vi "System_Host_2-1-2.vi"() -> ()   [LabVIEW 2017]
uses:
  <vilib>/Analysis/baseanly.llb/Mean (DBL).vi
  <vilib>/Utility/file.llb/Read Delimited Spreadsheet (string).vi
  <vilib>/Utility/file.llb/Write Delimited Spreadsheet (string).vi
  <vilib>/Utility/file.llb/Read Delimited Spreadsheet (DBL).vi
  <vilib>/Utility/file.llb/Write Delimited Spreadsheet (DBL).vi
  <resource>/objmgr/ni.dex.rc
  <vilib>/Analysis/NI_AALBase.lvlib
panel:
  out "System Time [s]":sgl
  out "Power Output":dbl(graph)
  out "Frequency [Hz]":u16(slide) scale=0.0..60.0
  out "Frequency [Hz]":u16(slide) scale=0.0..60.0
  out "Frequency [Hz]":u16(knob) scale=0.0..23.0
  out "Power [W]":dbl(slide) caption="Power Output [W]" scale=0.0..10000.0
  in  "Desired Power [W]":dbl
  out "WT-10":sgl format="%.1g"
  out "BT-11":sgl format="%.1g"
  out "BT-12":sgl format="%.1g"
  out "WT-13":sgl format="%.1g"
  out "CX-10":dbl format="%.1g"
  out "CX-11":dbl format="%.1g"
  out "WT-20":sgl format="%.1f"
  out "BT-21":sgl format="%.1f"
  out "WT-22":sgl format="%.1f"
  out "BT-23":sgl format="%.1f"
  out "WT-24":sgl format="%.1f"
  out "BT-25":sgl format="%.1f"
  out "WT-26":sgl format="%.1f"
  out "BT-27":sgl format="%.1f"
  out "WT-28":sgl format="%.1f"
  out "BT-29":sgl format="%.1f"
  out "BT-30":sgl format="%.1g"
  out "WT-31":sgl format="%.1g"
  out "BT-32":sgl format="%.1g"
  out "WT-33":sgl format="%.1g"
  out "BT-34":sgl format="%.1g"
  out "WT-35":sgl format="%.1g"
  out "WT-40":sgl format="%.1g"
  out "BT-41":sgl format="%.1g"
  out "WT-42":sgl format="%.1g"
  out "BT-43":sgl format="%.1g"
  out "BT-60":sgl format="%.1f"
  out "WT-61":sgl format="%.1f"
  out "WT-62":sgl format="%.1f"
  out "BT-63":sgl format="%.1f"
  out "WT-64":sgl format="%.1f"
  out "BT-65":sgl format="%.1f"
  out "BT-66":sgl format="%.1f"
  out "WT-67":sgl format="%.1f"
  out "ST-10":sgl format="%.1g"
  out "ST-11":sgl format="%.1g"
  out "ST-12":sgl[](array[numeric]) format="%.1g"
  out "ST-13":sgl format="%.1g"
  out "ST-14":sgl[](array[numeric]) format="%.1g"
  out "AT-01":sgl format="%.1g"
  out "AT-02":sgl format="%.1g"
  in  "Power Output On":bool
  in  "Shutdown":bool
  in  "ACTIVATE - CTAH":bool
  in  "CTAH Frequency [Hz]":u16
  in  "ACTIVATE - TCHX":bool
  in  "TCHX Frequency [Hz]":u16
  in  "ACTIVATE - PUMP":bool
  in  "Pump Frequency [Hz]":u16
  out "DHX Primary Flow\n\n\nFM-20 [kg/s]":sgl format="%.3f"
  out "Bypass Flow\n\n\nFM-30 [kg/s]":sgl format="%.3f"
  out "Primary Flow\n\n\nFM-40 [kg/s]":sgl format="%.3f"
  out "DRACS Flow\n\n\nFM-60 [kg/s]":sgl format="%.3f"
  in  "Flow Data?":bool=TRUE
  out "System Safe":bool
  in  "Exit Profile":bool
  in  "Select Operation Mode":T1(ring) caption="Select Operation Mode2"
  out "System Loop Time (ms)":u32
  in  "Load Power Profile":bool
  in  "Dyn. Power Profile File":path
  out "CTAH Temperatures":cluster{"CTAH Outlet":dbl, "CTAH Inlet":dbl}(graph)
  out "CTAH Outlet":dbl format="%0.2f"
  out "CTAH Inlet":dbl format="%0.2f"
  out "Core Temperatures":cluster{"Heater Inlet":dbl, "Heater Outlet":dbl}(graph)
  out "Heater Outlet":dbl format="%0.2f"
  out "Heater Inlet":dbl format="%0.2f"
  out "Profile Step":i32
  out "Power Input Signal [W]":dbl
  out "Output Current 2 [A]":dbl
  out "Output Voltage 2 [V]":dbl
  out "Output Current 1 [A]":dbl
  out "Output Voltage 1 [V]":dbl
  out "Loop Period [ms]":i64
  in  "Pump Operation Mode":i32(listbox)
  in  "TCHX Operation Mode":i32(listbox)
  in  "VFD Stop":bool
  in  "CTAH Operation Mode":i32(listbox)
  in  "Error In":errorcluster
  out "Number of Disconnections":u32
  out "Available Elements for Reading":i32
  out "DAQ?":bool
  in  "Stop DAQ":bool
  out "Error Out":errorcluster
  # "DRACS"
  # "PRIMARY"
  # "HOT DRACS"
  # "HOT LEG"
  # "DHX TOP"
  # "COLD DRACS"
  # "DHX"
  # "BYPASS"
  # "DHX BOTTOM"
  # "COLD LEG"
  # "PUMP"
  # "TCHX"
  # "CTAH"
  # "HEATER"
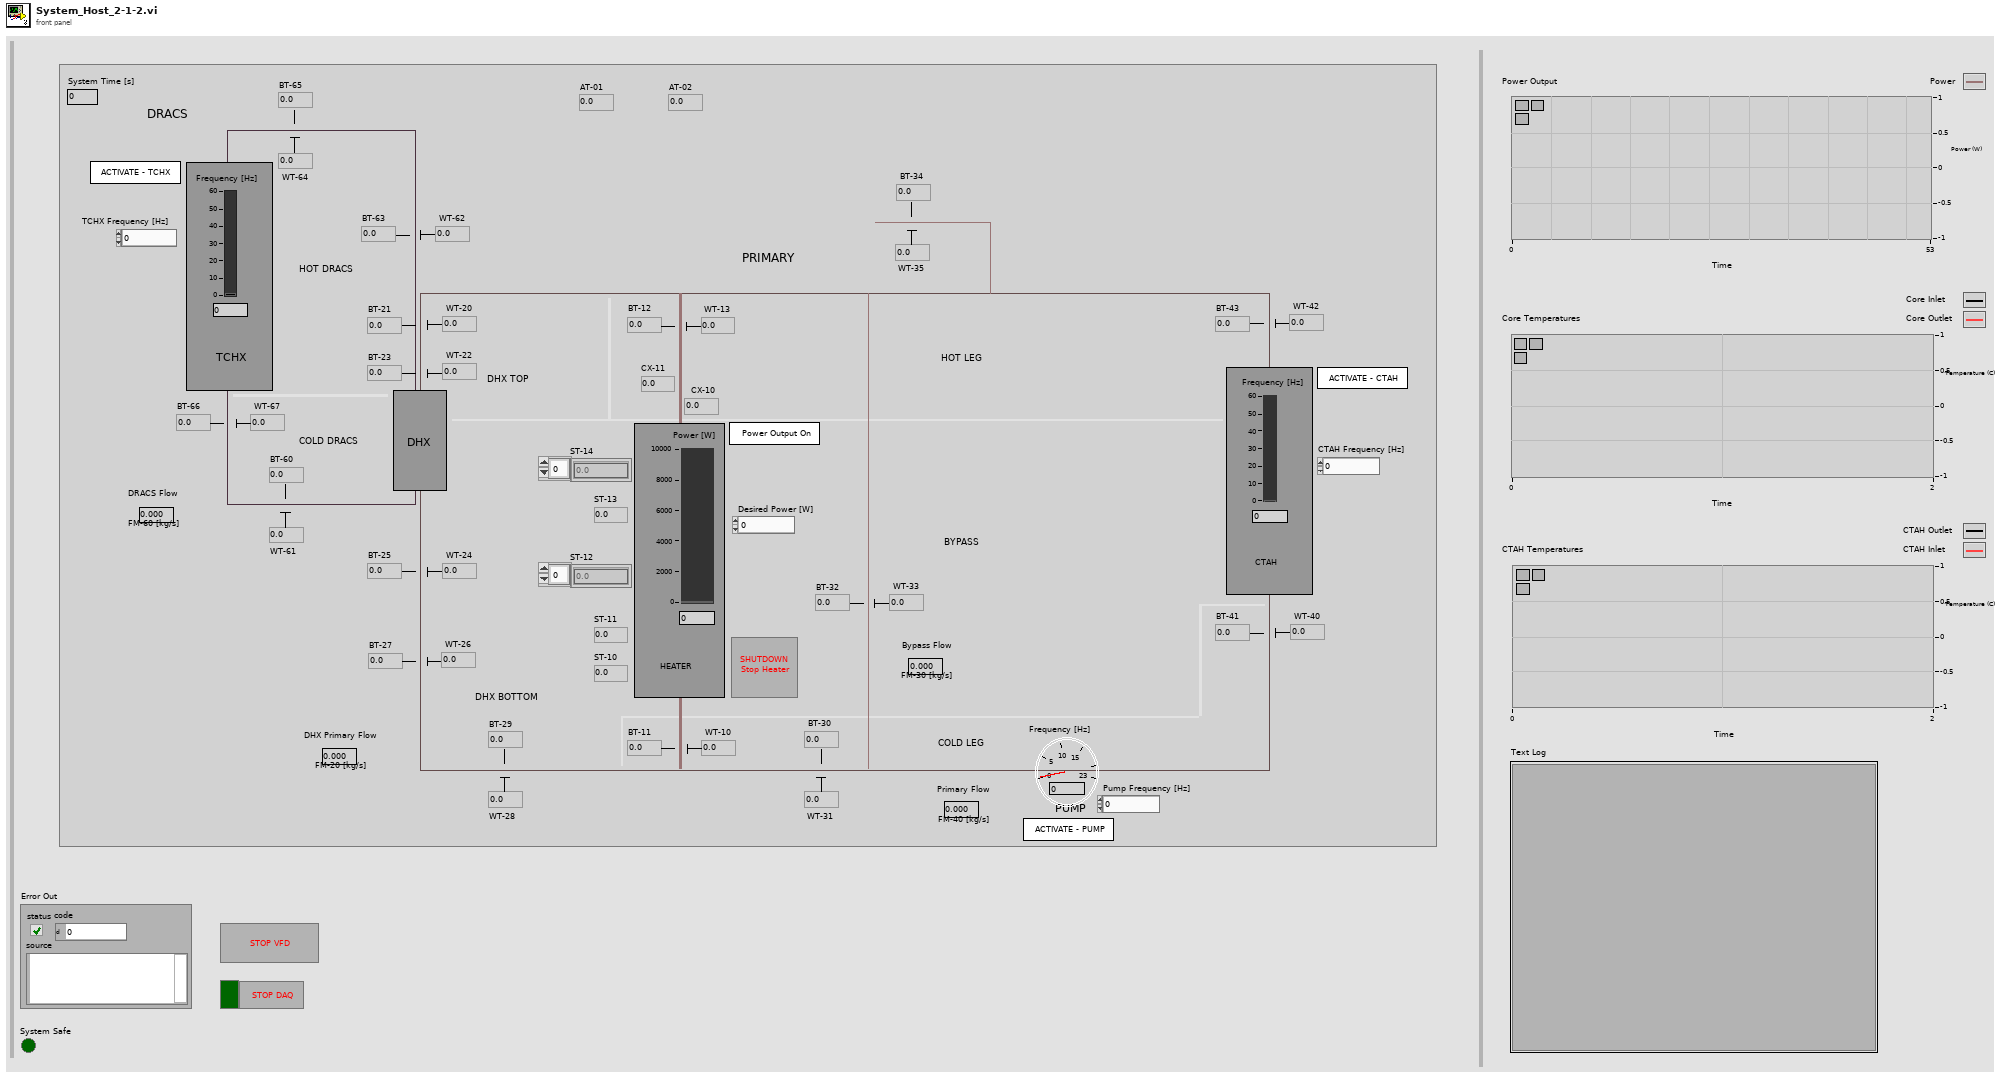
[diagram p1: front panel]
types:
  T1 = enum16{"Resistance Feedback", "Power Profile Input", "Resistance Feedback_Analog", "Power Profile Input_Analog", "Shutdown"}
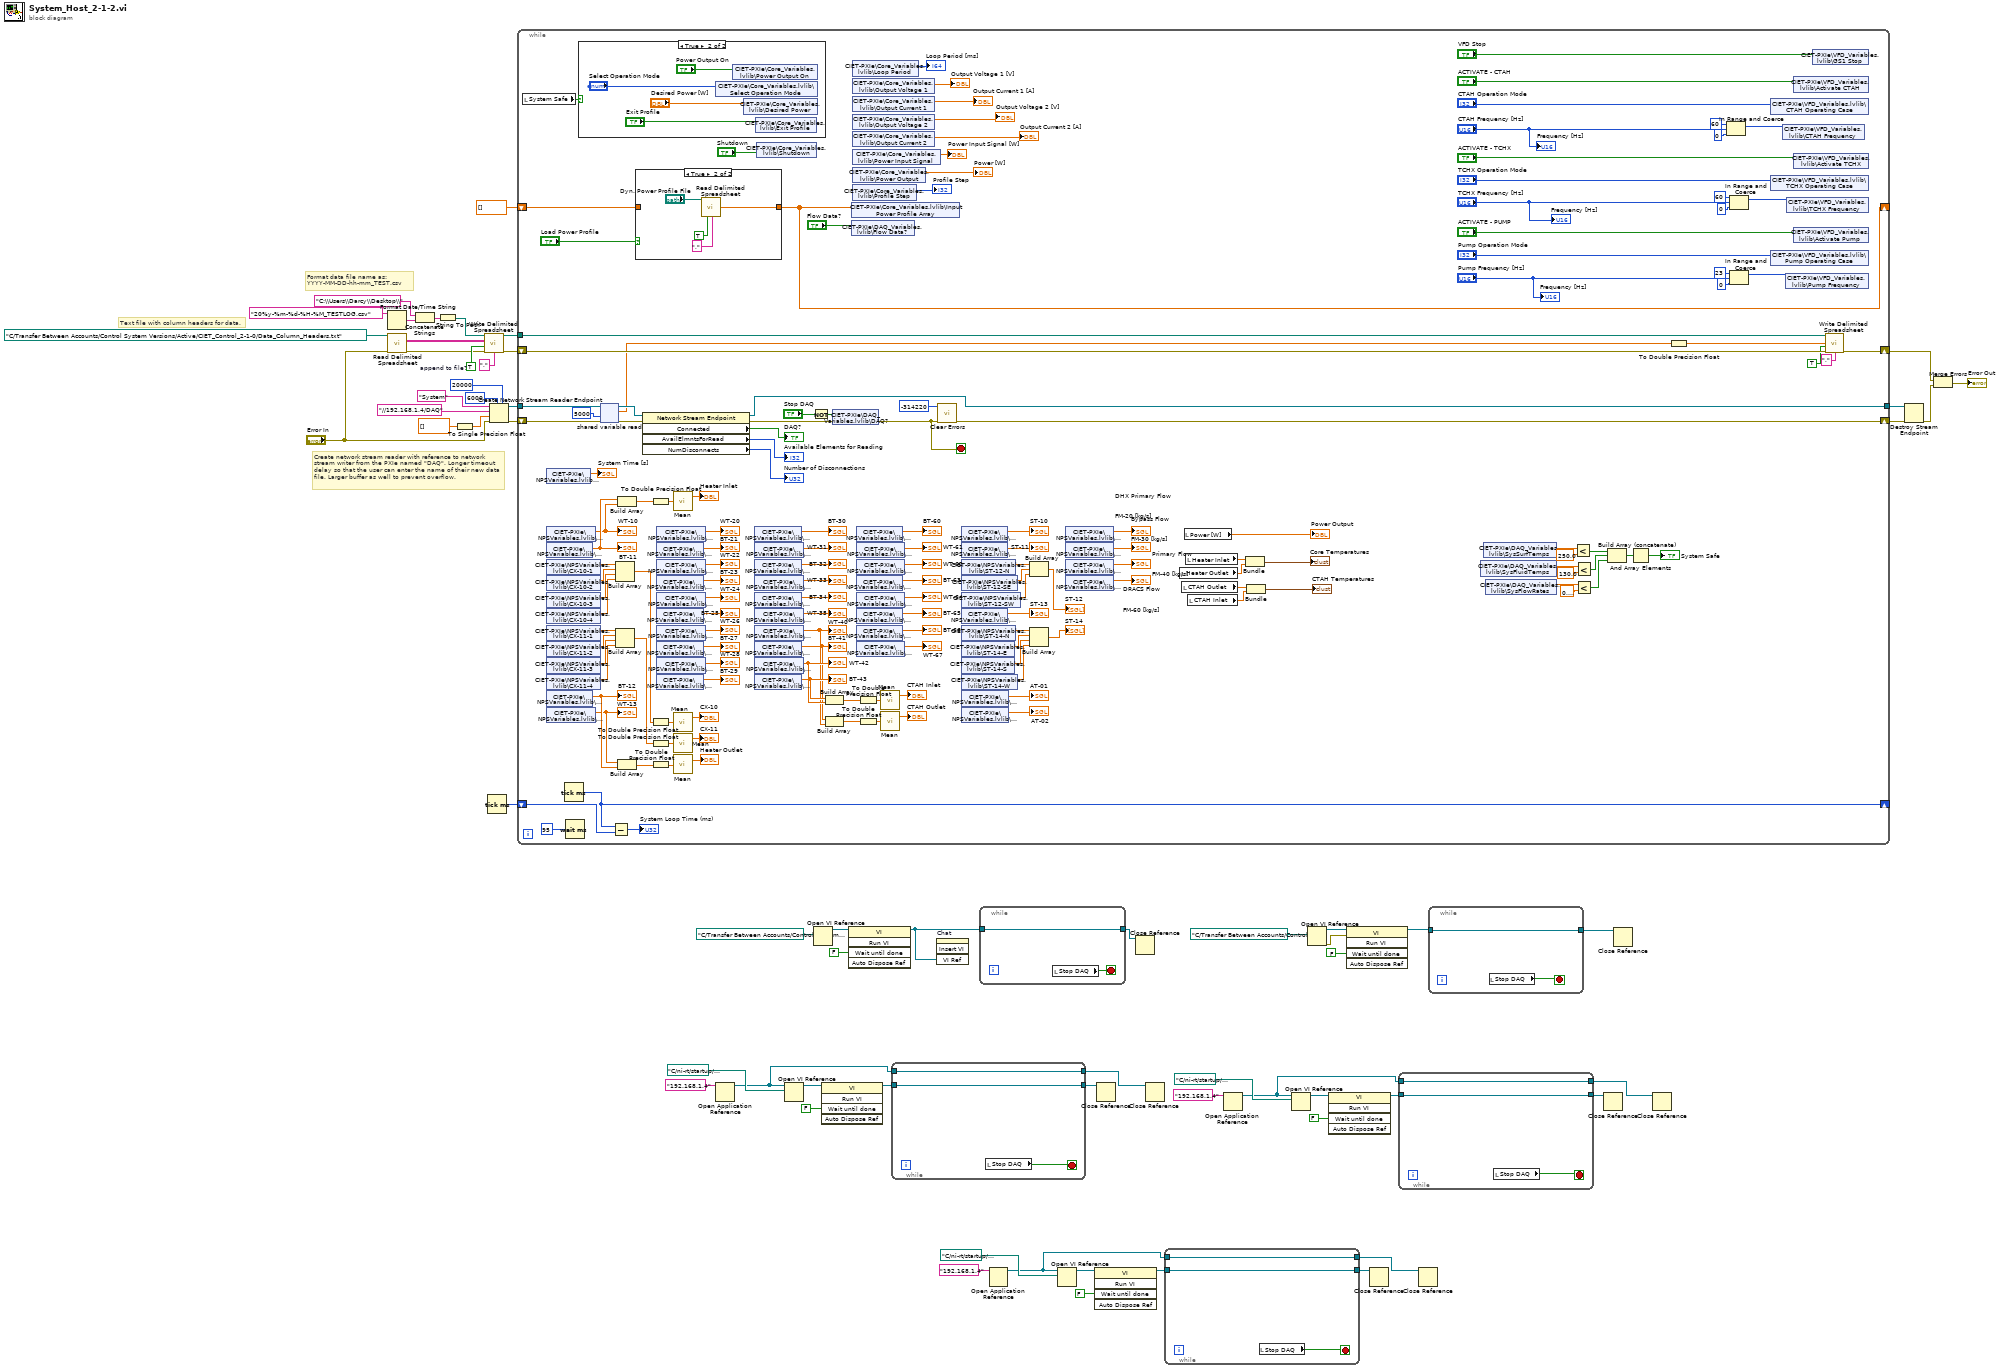
[diagram p0: block diagram]
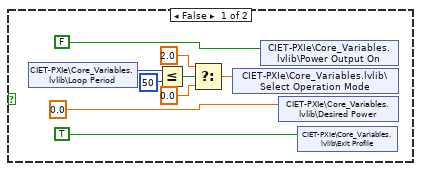
[diagram p2: hidden frame]
diagram:
  w50 = TRUE  # append to file?
  # "Format data file name as:\nYYYY-MM-DD-hh-mm_TEST.csv"
  # "Create network stream reader with reference to network\nstream writer from the PXIe named \"DAQ\". Longer timeout\ndelay so that the user can enter the name of their new data\nfile. Larger buffer as well to prevent overflow."
  # "Text file with column headers for data."
  n1 = Format Date/Time String(time format string (%c)="20%y-%m-%d-%H-%M_TESTLOG.csv") -> (date/time string=w40:string)  [unwired: 2 in]
  n2 = call-poly <vilib>:"Read Delimited Spreadsheet.vi"("file path (dialog if empty)"=path "C:/Transfer Between Accounts/Control System Versions/Active/CIET_Control_2-1-0/Data_Column_Headers.txt", "error in (no error)"="Error In") -> ("all rows"=w53:string[][], "error out"=w48:errorcluster)  [unwired: 8 in, 4 out]
  n3 = Concatenate Strings("C:\\Users\\Darcy\\Desktop\\" ("string"), w40) -> (w42:string)
  n4 = String To Path(string=w42) -> (path=w39:path)
  n5 = To Single Precision Float(number=dbl[] []) -> (single precision float=w61:sgl[])
  n6 = call-poly <vilib>:"Write Delimited Spreadsheet.vi"("file path (dialog if empty)"=w39, "2D data"=w53, "append to file? (new file:F)"=w50, "error in (no error)"=w48, "delimiter (\\t)"=",") -> ("new file path (Not A Path if cancelled)"=w49:path, "error out"=w47:errorcluster)  [unwired: 9 in]
  n7 = Tick Count (ms)() -> (millisecond timer value=w36:u32)
  n8 = Create Network Stream Reader Endpoint(5:20000 ("timeout in ms (-1)"), 7:6000 ("reader buffer size"), 8:"Error In", 9:w61, 10:"//192.168.1.4/DAQ" ("writer url"), 11:"System" ("reader name")) -> (0:w58:errorcluster, 3:w57:refnum<k21>)  [unwired: 1 in]
  n9 = while {
    shift-right: [w206] -> w56
    shift-left: w58 -> [w214]
    tunnel: w57 -> [w215]
    tunnel: [w205] -> w55
    tunnel: w49 -> [w201]
    shift-right: [w199] -> w46
    shift-left: w47 -> [w200]
    shift-right: [w89] -> _
    shift-left: dbl[] [] ("Input Power Profile Array") -> [w90]
    shift-right: [w86] -> _
    shift-left: w36 -> [w87]
    stop <- w204 stop-if-true
    n10 = local read "System Safe"() -> (w69:bool)
    n11 = shared-variable "CIET-PXIe\\NPSVariables.lvlib\\Time"() -> (→"System Time [s]":sgl)  [unwired: 1 in, 1 out]
    n12 = shared-variable "CIET-PXIe\\NPSVariables.lvlib\\WT-10"() -> (w110:sgl)  [unwired: 1 in, 1 out]
    "WT-10" <- w110
    n13 = shared-variable "CIET-PXIe\\NPSVariables.lvlib\\BT-11"() -> (w111:sgl)  [unwired: 1 in, 1 out]
    "BT-11" <- w111
    n14 = shared-variable "CIET-PXIe\\NPSVariables.lvlib\\CX-10-1"() -> (w173:sgl)  [unwired: 1 in, 1 out]
    n15 = shared-variable "CIET-PXIe\\NPSVariables.lvlib\\CX-10-2"() -> (w172:sgl)  [unwired: 1 in, 1 out]
    n16 = shared-variable "CIET-PXIe\\NPSVariables.lvlib\\CX-10-3"() -> (w171:sgl)  [unwired: 1 in, 1 out]
    n17 = shared-variable "CIET-PXIe\\NPSVariables.lvlib\\CX-10-4"() -> (w170:sgl)  [unwired: 1 in, 1 out]
    n18 = shared-variable "CIET-PXIe\\NPSVariables.lvlib\\CX-11-1"() -> (w166:sgl)  [unwired: 1 in, 1 out]
    n19 = shared-variable "CIET-PXIe\\NPSVariables.lvlib\\CX-11-2"() -> (w165:sgl)  [unwired: 1 in, 1 out]
    n20 = shared-variable "CIET-PXIe\\NPSVariables.lvlib\\CX-11-3"() -> (w164:sgl)  [unwired: 1 in, 1 out]
    n21 = shared-variable "CIET-PXIe\\NPSVariables.lvlib\\CX-11-4"() -> (w163:sgl)  [unwired: 1 in, 1 out]
    n22 = shared-variable "CIET-PXIe\\NPSVariables.lvlib\\BT-12"() -> (w115:sgl)  [unwired: 1 in, 1 out]
    "BT-12" <- w115
    n23 = shared-variable "CIET-PXIe\\NPSVariables.lvlib\\WT-13"() -> (w114:sgl)  [unwired: 1 in, 1 out]
    "WT-13" <- w114
    n24 = Tick Count (ms)() -> (millisecond timer value=w86:u32)
    n25 = Wait (ms)(milliseconds to wait=u32 95) -> ()  [unwired: 1 out]
    n26 = case shown="True" w69 {
      frame False {
        n27 = shared-variable "CIET-PXIe\\Core_Variables.lvlib\\Loop Period"() -> (w222:i64)  [unwired: 1 in, 1 out]
        n28 = Less Or Equal?(x=w222, y=i64 50) -> (x <= y?=w223:bool)
        n29 = Select(t=2.0, s=w223, f=0.0) -> (s? t:f=w218:dbl)
        n30 = shared-variable "CIET-PXIe\\Core_Variables.lvlib\\Select Operation Mode"(w218) -> ()  [unwired: 1 in, 1 out]
        n31 = shared-variable "CIET-PXIe\\Core_Variables.lvlib\\Power Output On"(FALSE ("Power Output On")) -> ()  [unwired: 1 in, 1 out]
        n32 = shared-variable "CIET-PXIe\\Core_Variables.lvlib\\Desired Power"(0.0 ("Desired Power")) -> ()  [unwired: 1 in, 1 out]
        n33 = shared-variable "CIET-PXIe\\Core_Variables.lvlib\\Exit Profile"(TRUE ("Exit Profile")) -> ()  [unwired: 1 in, 1 out]
      }
      frame True {
        n34 = shared-variable "CIET-PXIe\\Core_Variables.lvlib\\Select Operation Mode"("Select Operation Mode") -> ()  [unwired: 1 in, 1 out]
        n35 = shared-variable "CIET-PXIe\\Core_Variables.lvlib\\Power Output On"("Power Output On") -> ()  [unwired: 1 in, 1 out]
        n36 = shared-variable "CIET-PXIe\\Core_Variables.lvlib\\Desired Power"("Desired Power [W]") -> ()  [unwired: 1 in, 1 out]
        n37 = shared-variable "CIET-PXIe\\Core_Variables.lvlib\\Exit Profile"("Exit Profile") -> ()  [unwired: 1 in, 1 out]
      }
    }
    n38 = shared-variable-read(w215, w214, 5000 ("timeout ms (-1)")) -> (w211:refnum<k21>, w209:errorcluster, w174:sgl[])  [unwired: 1 out]
    n39 = Subtract(x=w86, y=w87) -> (x-y=→"System Loop Time (ms)":u32)
    n40 = Build Array(w173, w172, w171, w170) -> (w169:sgl[])
    n41 = Build Array(w166, w165, w164, w163) -> (w162:sgl[])
    n42 = Build Array(w111, w110) -> (w112:sgl[])
    n43 = Build Array(w114, w115) -> (w116:sgl[])
    n44 = case shown="True" "Load Power Profile" {
      tunnel: [w231 w232] -> w89
      tunnel: w90 -> [w231 _]
      frame False {
      }
      frame True {
        n45 = call-poly <vilib>:"Read Delimited Spreadsheet.vi"("file path (dialog if empty)"="Dyn. Power Profile File", "transpose? (F)"=TRUE, "delimiter (\\t)"="," ("delimiter (\\t)")) -> ("first row"=w232:dbl[])  [unwired: 7 in, 5 out]
      }
    }
    n46 = property class="Network Stream Endpoint"(reference=w211, error in=w209) -> (reference out=w205:refnum<k21>, error out=w210:errorcluster, "Connected"=→"DAQ?":bool, "AvailElmntsForRead"=→"Available Elements for Reading":i32, "NumDisconnects"=→"Number of Disconnections":u32)
    n47 = To Double Precision Float(number=w112) -> (double precision float=w113:dbl[])
    n48 = To Double Precision Float(number=w169) -> (double precision float=w168:dbl[])
    n49 = To Double Precision Float(number=w162) -> (double precision float=w167:dbl[])
    n50 = To Double Precision Float(number=w116) -> (double precision float=w117:dbl[])
    n51 = shared-variable "CIET-PXIe\\NPSVariables.lvlib\\WT-20"() -> (→"WT-20":sgl)  [unwired: 1 in, 1 out]
    n52 = shared-variable "CIET-PXIe\\NPSVariables.lvlib\\BT-21"() -> (→"BT-21":sgl)  [unwired: 1 in, 1 out]
    n53 = shared-variable "CIET-PXIe\\NPSVariables.lvlib\\WT-22"() -> (→"WT-22":sgl)  [unwired: 1 in, 1 out]
    n54 = shared-variable "CIET-PXIe\\NPSVariables.lvlib\\BT-23"() -> (→"BT-23":sgl)  [unwired: 1 in, 1 out]
    n55 = shared-variable "CIET-PXIe\\NPSVariables.lvlib\\WT-24"() -> (→"WT-24":sgl)  [unwired: 1 in, 1 out]
    n56 = shared-variable "CIET-PXIe\\NPSVariables.lvlib\\BT-25"() -> (→"BT-25":sgl)  [unwired: 1 in, 1 out]
    n57 = shared-variable "CIET-PXIe\\NPSVariables.lvlib\\WT-26"() -> (→"WT-26":sgl)  [unwired: 1 in, 1 out]
    n58 = shared-variable "CIET-PXIe\\NPSVariables.lvlib\\BT-27"() -> (→"BT-27":sgl)  [unwired: 1 in, 1 out]
    n59 = shared-variable "CIET-PXIe\\NPSVariables.lvlib\\WT-28"() -> (→"WT-28":sgl)  [unwired: 1 in, 1 out]
    n60 = shared-variable "CIET-PXIe\\NPSVariables.lvlib\\BT-29"() -> (→"BT-29":sgl)  [unwired: 1 in, 1 out]
    n61 = call-poly <vilib>:"Mean.vi"("X"=w113) -> ("mean"=→"Heater Inlet":dbl)  [unwired: 1 out]
    n62 = call-poly <vilib>:"Mean.vi"("X"=w168) -> ("mean"=→"CX-10":dbl)  [unwired: 1 out]
    n63 = call-poly <vilib>:"Mean.vi"("X"=w167) -> ("mean"=→"CX-11":dbl)  [unwired: 1 out]
    n64 = call-poly <vilib>:"Mean.vi"("X"=w117) -> ("mean"=→"Heater Outlet":dbl)  [unwired: 1 out]
    n65 = shared-variable "CIET-PXIe\\NPSVariables.lvlib\\BT-30"() -> (→"BT-30":sgl)  [unwired: 1 in, 1 out]
    n66 = shared-variable "CIET-PXIe\\NPSVariables.lvlib\\WT-31"() -> (→"WT-31":sgl)  [unwired: 1 in, 1 out]
    n67 = shared-variable "CIET-PXIe\\NPSVariables.lvlib\\BT-32"() -> (→"BT-32":sgl)  [unwired: 1 in, 1 out]
    n68 = shared-variable "CIET-PXIe\\NPSVariables.lvlib\\WT-33"() -> (→"WT-33":sgl)  [unwired: 1 in, 1 out]
    n69 = shared-variable "CIET-PXIe\\NPSVariables.lvlib\\BT-34"() -> (→"BT-34":sgl)  [unwired: 1 in, 1 out]
    n70 = shared-variable "CIET-PXIe\\NPSVariables.lvlib\\WT-35"() -> (→"WT-35":sgl)  [unwired: 1 in, 1 out]
    n71 = shared-variable "CIET-PXIe\\NPSVariables.lvlib\\WT-40"() -> (w96:sgl)  [unwired: 1 in, 1 out]
    "WT-40" <- w96
    n72 = shared-variable "CIET-PXIe\\NPSVariables.lvlib\\BT-41"() -> (w95:sgl)  [unwired: 1 in, 1 out]
    "BT-41" <- w95
    n73 = shared-variable "CIET-PXIe\\NPSVariables.lvlib\\WT-42"() -> (w98:sgl)  [unwired: 1 in, 1 out]
    "WT-42" <- w98
    n74 = shared-variable "CIET-PXIe\\NPSVariables.lvlib\\BT-43"() -> (w97:sgl)  [unwired: 1 in, 1 out]
    "BT-43" <- w97
    n75 = shared-variable "CIET-PXIe\\Core_Variables.lvlib\\Shutdown"("Shutdown") -> ()  [unwired: 1 in, 1 out]
    n76 = Not(x="Stop DAQ") -> (.not. x?=w213:bool)
    n77 = Build Array(w97, w98) -> (w103:sgl[])
    n78 = Build Array(w95, w96) -> (w100:sgl[])
    n79 = shared-variable "CIET-PXIe\\DAQ_Variables.lvlib\\DAQ?"(w213, error in=w210) -> (error out=w204:errorcluster)
    n80 = shared-variable "CIET-PXIe\\Core_Variables.lvlib\\Input Power Profile Array"(w89) -> ()  [unwired: 1 in, 1 out]
    n81 = shared-variable "CIET-PXIe\\DAQ_Variables.lvlib\\Flow Data?"("Flow Data?") -> ()  [unwired: 1 in, 1 out]
    n82 = shared-variable "CIET-PXIe\\Core_Variables.lvlib\\Loop Period"() -> (→"Loop Period [ms]":i64)  [unwired: 1 in, 1 out]
    n83 = shared-variable "CIET-PXIe\\Core_Variables.lvlib\\Output Voltage 1"() -> (→"Output Voltage 1 [V]":dbl)  [unwired: 1 in, 1 out]
    n84 = shared-variable "CIET-PXIe\\Core_Variables.lvlib\\Output Current 1"() -> (→"Output Current 1 [A]":dbl)  [unwired: 1 in, 1 out]
    n85 = shared-variable "CIET-PXIe\\Core_Variables.lvlib\\Output Voltage 2"() -> (→"Output Voltage 2 [V]":dbl)  [unwired: 1 in, 1 out]
    n86 = shared-variable "CIET-PXIe\\Core_Variables.lvlib\\Output Current 2"() -> (→"Output Current 2 [A]":dbl)  [unwired: 1 in, 1 out]
    n87 = shared-variable "CIET-PXIe\\Core_Variables.lvlib\\Power Input Signal"() -> (→"Power Input Signal [W]":dbl)  [unwired: 1 in, 1 out]
    n88 = shared-variable "CIET-PXIe\\Core_Variables.lvlib\\Power Output"() -> (→"Power [W]":dbl)  [unwired: 1 in, 1 out]
    n89 = shared-variable "CIET-PXIe\\Core_Variables.lvlib\\Profile Step"() -> (→"Profile Step":i32)  [unwired: 1 in, 1 out]
    n90 = shared-variable "CIET-PXIe\\NPSVariables.lvlib\\BT-60"() -> (→"BT-60":sgl)  [unwired: 1 in, 1 out]
    n91 = shared-variable "CIET-PXIe\\NPSVariables.lvlib\\WT-61"() -> (→"WT-61":sgl)  [unwired: 1 in, 1 out]
    n92 = shared-variable "CIET-PXIe\\NPSVariables.lvlib\\WT-62"() -> (→"WT-62":sgl)  [unwired: 1 in, 1 out]
    n93 = shared-variable "CIET-PXIe\\NPSVariables.lvlib\\BT-63"() -> (→"BT-63":sgl)  [unwired: 1 in, 1 out]
    n94 = shared-variable "CIET-PXIe\\NPSVariables.lvlib\\WT-64"() -> (→"WT-64":sgl)  [unwired: 1 in, 1 out]
    n95 = shared-variable "CIET-PXIe\\NPSVariables.lvlib\\BT-65"() -> (→"BT-65":sgl)  [unwired: 1 in, 1 out]
    n96 = shared-variable "CIET-PXIe\\NPSVariables.lvlib\\BT-66"() -> (→"BT-66":sgl)  [unwired: 1 in, 1 out]
    n97 = shared-variable "CIET-PXIe\\NPSVariables.lvlib\\WT-67"() -> (→"WT-67":sgl)  [unwired: 1 in, 1 out]
    n98 = To Double Precision Float(number=w103) -> (double precision float=w104:dbl[])
    n99 = To Double Precision Float(number=w100) -> (double precision float=w101:dbl[])
    n100 = call-poly <vilib>:"Mean.vi"("X"=w104) -> ("mean"=→"CTAH Inlet":dbl)  [unwired: 1 out]
    n101 = call-poly <vilib>:"Mean.vi"("X"=w101) -> ("mean"=→"CTAH Outlet":dbl)  [unwired: 1 out]
    n102 = call <vilib>:"Clear Errors.vi"("error in (no error)"=w204, "specific error code to clear (0: all)"=-314220) -> ("error out"=w206:errorcluster)  [unwired: 4 in, 1 out]
    n103 = shared-variable "CIET-PXIe\\NPSVariables.lvlib\\ST-10"() -> (→"ST-10":sgl)  [unwired: 1 in, 1 out]
    n104 = shared-variable "CIET-PXIe\\NPSVariables.lvlib\\ST-11"() -> (→"ST-11":sgl)  [unwired: 1 in, 1 out]
    n105 = shared-variable "CIET-PXIe\\NPSVariables.lvlib\\ST-12-N"() -> (w133:sgl)  [unwired: 1 in, 1 out]
    n106 = shared-variable "CIET-PXIe\\NPSVariables.lvlib\\ST-12-SE"() -> (w132:sgl)  [unwired: 1 in, 1 out]
    n107 = shared-variable "CIET-PXIe\\NPSVariables.lvlib\\ST-12-SW"() -> (w131:sgl)  [unwired: 1 in, 1 out]
    n108 = shared-variable "CIET-PXIe\\NPSVariables.lvlib\\ST-13"() -> (→"ST-13":sgl)  [unwired: 1 in, 1 out]
    n109 = shared-variable "CIET-PXIe\\NPSVariables.lvlib\\ST-14-N"() -> (w128:sgl)  [unwired: 1 in, 1 out]
    n110 = shared-variable "CIET-PXIe\\NPSVariables.lvlib\\ST-14-E"() -> (w127:sgl)  [unwired: 1 in, 1 out]
    n111 = shared-variable "CIET-PXIe\\NPSVariables.lvlib\\ST-14-S"() -> (w126:sgl)  [unwired: 1 in, 1 out]
    n112 = shared-variable "CIET-PXIe\\NPSVariables.lvlib\\ST-14-W"() -> (w125:sgl)  [unwired: 1 in, 1 out]
    n113 = shared-variable "CIET-PXIe\\NPSVariables.lvlib\\AT-01"() -> (→"AT-01":sgl)  [unwired: 1 in, 1 out]
    n114 = shared-variable "CIET-PXIe\\NPSVariables.lvlib\\AT-02"() -> (→"AT-02":sgl)  [unwired: 1 in, 1 out]
    n115 = Build Array(w133, w132, w131) -> (→"ST-12":sgl[])
    n116 = Build Array(w128, w127, w126, w125) -> (→"ST-14":sgl[])
    n117 = shared-variable "CIET-PXIe\\NPSVariables.lvlib\\FM-20"() -> (→"DHX Primary Flow\n\n\nFM-20 [kg/s]":sgl)  [unwired: 1 in, 1 out]
    n118 = shared-variable "CIET-PXIe\\NPSVariables.lvlib\\FM-30"() -> (→"Bypass Flow\n\n\nFM-30 [kg/s]":sgl)  [unwired: 1 in, 1 out]
    n119 = shared-variable "CIET-PXIe\\NPSVariables.lvlib\\FM-40"() -> (→"Primary Flow\n\n\nFM-40 [kg/s]":sgl)  [unwired: 1 in, 1 out]
    n120 = shared-variable "CIET-PXIe\\NPSVariables.lvlib\\FM-60"() -> (→"DRACS Flow\n\n\nFM-60 [kg/s]":sgl)  [unwired: 1 in, 1 out]
    n121 = local read "Heater Outlet"() -> (w105:dbl)
    n122 = local read "CTAH Outlet"() -> (w93:dbl)
    n123 = local read "Power [W]"() -> (→"Power Output":dbl)
    n124 = local read "Heater Inlet"() -> (w106:dbl)
    n125 = local read "CTAH Inlet"() -> (w92:dbl)
    n126 = Bundle("Heater Inlet"=w106, "Heater Outlet"=w105) -> (→"Core Temperatures":cluster{"Heater Inlet":dbl, "Heater Outlet":dbl})  [unwired: 1 in]
    n127 = Bundle("CTAH Outlet"=w93, "CTAH Inlet"=w92) -> (→"CTAH Temperatures":cluster{"CTAH Outlet":dbl, "CTAH Inlet":dbl})  [unwired: 1 in]
    n128 = shared-variable "CIET-PXIe\\DAQ_Variables.lvlib\\SysFluidTemps"() -> (w75:sgl[])  [unwired: 1 in, 1 out]
    n129 = shared-variable "CIET-PXIe\\DAQ_Variables.lvlib\\SysSurfTemps"() -> (w77:sgl[])  [unwired: 1 in, 1 out]
    n130 = shared-variable "CIET-PXIe\\DAQ_Variables.lvlib\\SysFlowRates"() -> (w73:sgl[])  [unwired: 1 in, 1 out]
    n131 = Less?(x=w77, y=sgl 250.0) -> (x < y?=w79:bool[])
    n132 = Less?(x=w75, y=sgl 130.0) -> (x < y?=w72:bool[])
    n133 = Less?(x=w73, y=sgl 0.2) -> (x < y?=w71:bool[])
    n134 = Build Array (concatenate)(w79, w72, w71) -> (w80:bool[])
    n135 = And Array Elements(Boolean array=w80) -> (logical AND=→"System Safe":bool)
    n136 = To Double Precision Float(number=w174) -> (double precision float=w88:dbl[])
    n137 = In Range and Coerce(upper limit=u16 60, x="CTAH Frequency [Hz]", lower limit=u16 0) -> (coerced(x)=w83:u16)  [unwired: 1 out]
    n138 = In Range and Coerce(upper limit=u16 60, x="TCHX Frequency [Hz]", lower limit=u16 0) -> (coerced(x)=w191:u16)  [unwired: 1 out]
    n139 = In Range and Coerce(upper limit=u16 23, x="Pump Frequency [Hz]", lower limit=u16 0) -> (coerced(x)=w186:u16)  [unwired: 1 out]
    n140 = shared-variable "CIET-PXIe\\VFD_Variables.lvlib\\CTAH Operating Case"("CTAH Operation Mode") -> ()  [unwired: 1 in, 1 out]
    n141 = shared-variable "CIET-PXIe\\VFD_Variables.lvlib\\Pump Operating Case"("Pump Operation Mode") -> ()  [unwired: 1 in, 1 out]
    n142 = shared-variable "CIET-PXIe\\VFD_Variables.lvlib\\TCHX Operating Case"("TCHX Operation Mode") -> ()  [unwired: 1 in, 1 out]
    n143 = shared-variable "CIET-PXIe\\VFD_Variables.lvlib\\CTAH Frequency"(w83) -> ()  [unwired: 1 in, 1 out]
    n144 = shared-variable "CIET-PXIe\\VFD_Variables.lvlib\\Pump Frequency"(w186) -> ()  [unwired: 1 in, 1 out]
    n145 = shared-variable "CIET-PXIe\\VFD_Variables.lvlib\\TCHX Frequency"(w191) -> ()  [unwired: 1 in, 1 out]
    n146 = shared-variable "CIET-PXIe\\VFD_Variables.lvlib\\Activate CTAH"("ACTIVATE - CTAH") -> ()  [unwired: 1 in, 1 out]
    n147 = shared-variable "CIET-PXIe\\VFD_Variables.lvlib\\Activate Pump"("ACTIVATE - PUMP") -> ()  [unwired: 1 in, 1 out]
    n148 = shared-variable "CIET-PXIe\\VFD_Variables.lvlib\\Activate TCHX"("ACTIVATE - TCHX") -> ()  [unwired: 1 in, 1 out]
    n149 = shared-variable "CIET-PXIe\\VFD_Variables.lvlib\\GS1 Stop"("VFD Stop") -> ()  [unwired: 1 in, 1 out]
    n150 = call-poly <vilib>:"Write Delimited Spreadsheet.vi"("file path (dialog if empty)"=w201, "1D data"=w88, "append to file? (new file:F)"=TRUE, "error in (no error)"=w200, "delimiter (\\t)"="," ("delimiter (\\t)")) -> ("error out"=w199:errorcluster)  [unwired: 9 in, 1 out]
    "Frequency [Hz]" <- "Pump Frequency [Hz]"
    "Frequency [Hz]" <- "CTAH Frequency [Hz]"
    "Frequency [Hz]" <- "TCHX Frequency [Hz]"
  }
  n151 = Open Application Reference(11:"192.168.1.4" ("machine name (\"\":  open local reference)")) -> (3:w23:refnum<vi>)  [unwired: 3 in, 1 out]
  n152 = Open VI Reference(application reference (local)=w23, vi path=path "C:/ni-rt/startup/DAQ.vi") -> (vi reference=w27:refnum<vi>)  [unwired: 4 in, 1 out]
  n153 = Open VI Reference(vi path=path "C:/Transfer Between Accounts/Control System Versions/Active/CIET_Control_2-1-0/Networking VIs/Updated Chat_Supervisor.vi") -> (vi reference=w4:refnum<vi>)  [unwired: 5 in, 1 out]
  n154 = invoke class="VI" method="Run VI"(reference=w27, "Wait until done"=FALSE ("Wait Until Done")) -> (reference out=w25:refnum<vi>)  [unwired: 3 in, 4 out]
  n155 = invoke class="VI" method="Run VI"(reference=w4, "Wait until done"=FALSE ("Wait Until Done")) -> (reference out=w2:refnum<vi>)  [unwired: 3 in, 4 out]
  n156 = while {
    tunnel: w25 -> [w237]
    tunnel: [w237] -> w24
    tunnel: w23 -> [w236]
    tunnel: [w236] -> w22
    stop <- w238 stop-if-true
    n157 = local read "Stop DAQ"() -> (w238:bool)
  }
  n158 = invoke on="Chat" class="SubPnl" method="Insert VI"("VI Ref"=w2) -> ()  [unwired: 3 in, 4 out]
  n159 = while {
    tunnel: w2 -> [w239]
    tunnel: [w239] -> w1
    stop <- w240 stop-if-true
    n160 = local read "Stop DAQ"() -> (w240:bool)
  }
  n161 = Open Application Reference(11:"192.168.1.4" ("machine name (\"\":  open local reference)")) -> (3:w7:refnum<vi>)  [unwired: 3 in, 1 out]
  n162 = Open VI Reference(application reference (local)=w7, vi path=path "C:/ni-rt/startup/VFD.vi") -> (vi reference=w11:refnum<vi>)  [unwired: 4 in, 1 out]
  n163 = invoke class="VI" method="Run VI"(reference=w11, "Wait until done"=FALSE ("Wait Until Done")) -> (reference out=w9:refnum<vi>)  [unwired: 3 in, 4 out]
  n164 = Close Reference(reference=w24) -> ()  [unwired: 1 in, 1 out]
  n165 = Close Reference(reference=w1) -> ()  [unwired: 1 in, 1 out]
  n166 = Close Reference(reference=w22) -> ()  [unwired: 1 in, 1 out]
  n167 = while {
    tunnel: w9 -> [w242]
    tunnel: [w242] -> w8
    tunnel: w7 -> [w241]
    tunnel: [w241] -> w6
    stop <- w243 stop-if-true
    n168 = local read "Stop DAQ"() -> (w243:bool)
  }
  n169 = Open Application Reference(11:"192.168.1.4" ("machine name (\"\":  open local reference)")) -> (3:w15:refnum<vi>)  [unwired: 3 in, 1 out]
  n170 = Open VI Reference(application reference (local)=w15, vi path=path "C:/ni-rt/startup/Core.vi") -> (vi reference=w19:refnum<vi>)  [unwired: 4 in, 1 out]
  n171 = Open VI Reference(vi path=path "C:/Transfer Between Accounts/Control System Versions/Active/CIET_Control_2-1-0/Networking VIs/OPC UA Server_String.vi") -> (vi reference=w32:refnum<vi>, error out=w35:errorcluster)  [unwired: 5 in]
  n172 = invoke class="VI" method="Run VI"(reference=w19, "Wait until done"=FALSE ("Wait Until Done")) -> (reference out=w17:refnum<vi>)  [unwired: 3 in, 4 out]
  n173 = invoke class="VI" method="Run VI"(reference=w32, error in=w35, "Wait until done"=FALSE ("Wait Until Done")) -> (reference out=w33:refnum<vi>)  [unwired: 2 in, 4 out]
  n174 = Close Reference(reference=w8) -> ()  [unwired: 1 in, 1 out]
  n175 = while {
    tunnel: w17 -> [w245]
    tunnel: [w245] -> w16
    tunnel: w15 -> [w244]
    tunnel: [w244] -> w14
    stop <- w246 stop-if-true
    n176 = local read "Stop DAQ"() -> (w246:bool)
  }
  n177 = Close Reference(reference=w6) -> ()  [unwired: 1 in, 1 out]
  n178 = while {
    tunnel: w33 -> [w248]
    tunnel: [w248] -> w34
    stop <- w247 stop-if-true
    n179 = local read "Stop DAQ"() -> (w247:bool)
  }
  n180 = Close Reference(reference=w16) -> ()  [unwired: 1 in, 1 out]
  n181 = Close Reference(reference=w34) -> ()  [unwired: 1 in, 1 out]
  n182 = Close Reference(reference=w14) -> ()  [unwired: 1 in, 1 out]
  n183 = Destroy Stream Endpoint(8:w56, 11:w55) -> (0:w45:errorcluster)
  n184 = Merge Errors(w46, w45) -> (→"Error Out":errorcluster)
